vi "Digital Pattern Gen 1.3 In Place Settings Write Structure.vi"(5 "device inputs":dbl[](array[numeric]), 6 "device outputs in":dbl[](array[numeric]), 7 "last device inputs":dbl[](array[numeric]), 8 "error in (no error)":errorcluster, 9 "FPGA ref in":T1, 11 "1.3 digital pattern gen in":T2) -> (0 "error out":errorcluster, 1 "FPGA ref out":T1, 3 "1.3 digital pattern gen out":T2, 4 "device outputs out":dbl[](array[numeric]))   [LabVIEW 2019, in "Engine Simulation Toolkit Engine.lvlib"]
uses:
  Engine Simulation Toolkit Engine.lvlib
  Shared/1.3 Digital Pattern Gen Engine Data.ctl
  Shared/1.3 Digital Pattern Gen FIFO Idxs.ctl
  Digital Pattern Gen 1.3 Settings Ref.ctl
  Shared/Engine Simulation Toolkit Shared.lvlib
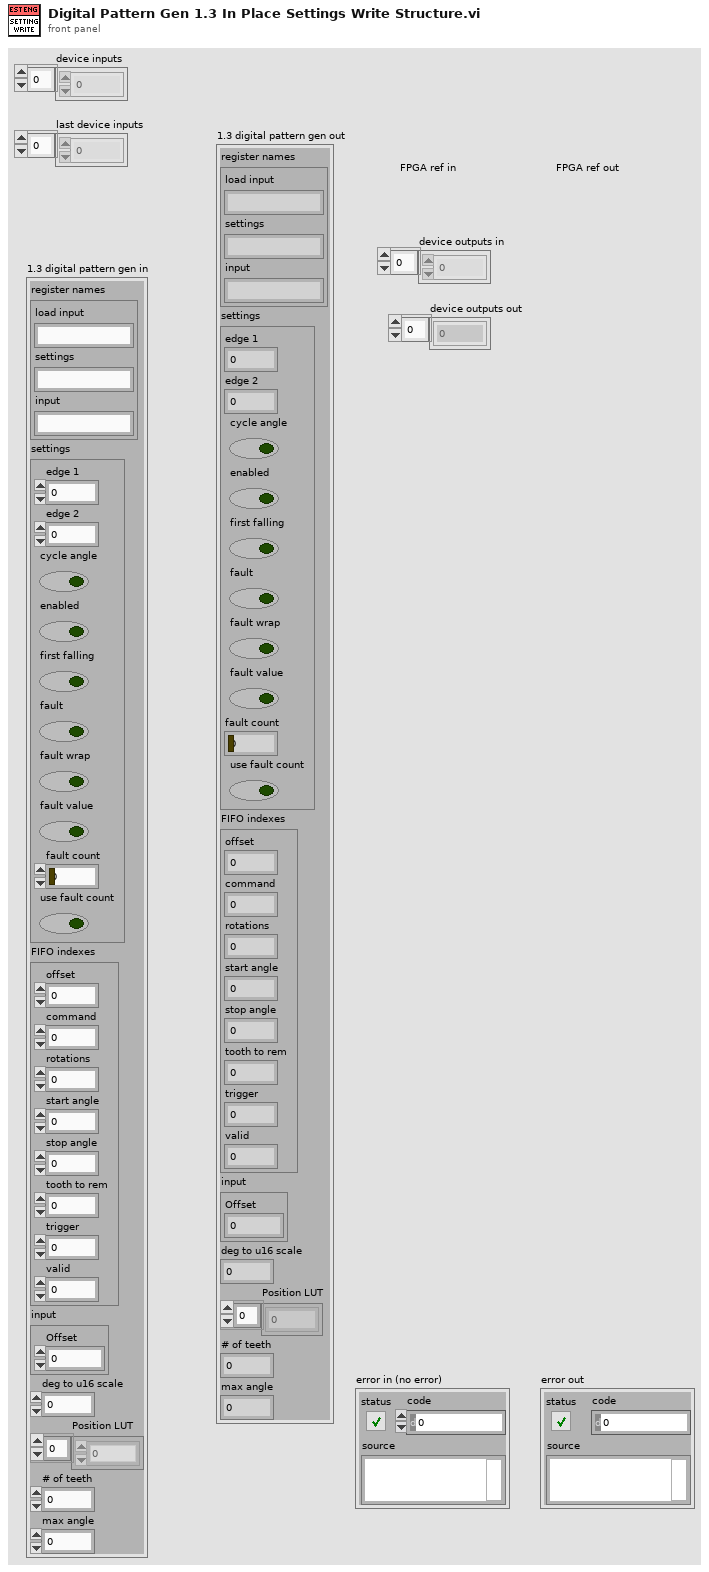
[diagram p1: front panel]
types:
  T1 = typedef "Engine Simulation Toolkit Engine.lvlib/Digital Pattern Gen 1.3 Settings Ref.ctl" = refnum<k20>
  T2 = typedef "Engine Simulation Toolkit Shared.lvlib/1.3 Digital Pattern Gen Engine Data.ctl" = cluster{"register names":cluster{"load input":string, "settings":string, "input":string}, "settings":cluster{"edge 1":u16, "edge 2":u16, "cycle angle":bool, "enabled":bool, "first falling":bool, "fault":bool, "fault wrap":bool, "fault value":bool, "fault count":fxp<+,4,4>, "use fault count":bool}, "FIFO indexes":T3, "input":cluster{"Offset":i16}, "deg to u16 scale":dbl, "Position LUT":u16[], "# of teeth":i16, "max angle":dbl}
  T3 = typedef "Engine Simulation Toolkit Shared.lvlib/1.3 Digital Pattern Gen FIFO Idxs.ctl" = cluster{"offset":i32, "command":i32, "rotations":i32, "start angle":i32, "stop angle":i32, "tooth to rem":i32, "trigger":i32, "valid":i32}
  T4 = cluster{"edge 1":u16, "edge 2":u16, "cycle angle":bool, "enabled":bool, "first falling":bool, "fault":bool, "fault wrap":bool, "fault value":bool, "fault count":fxp<+,4,4>, "use fault count":bool}
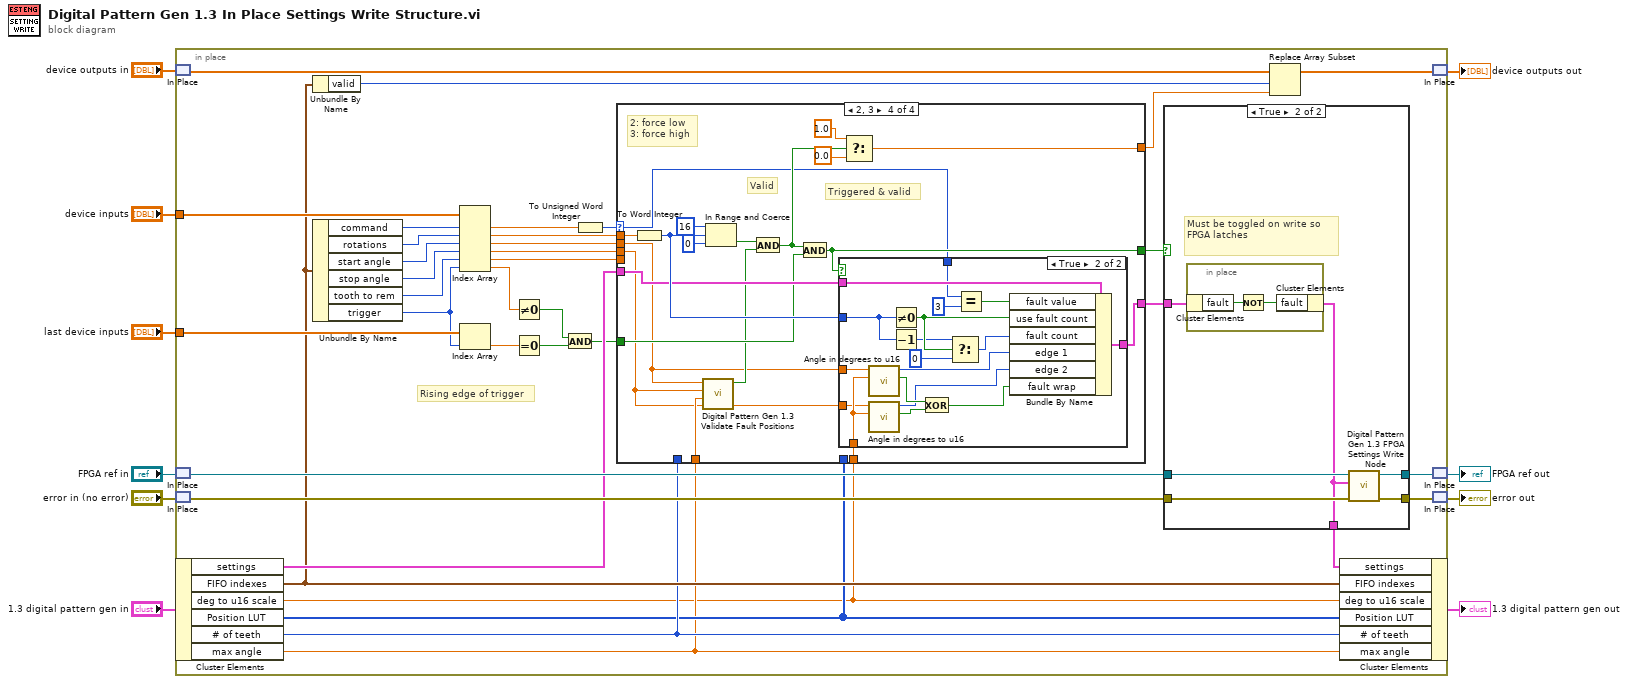
[diagram p0: block diagram]
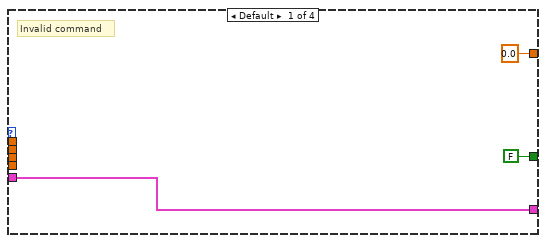
[diagram p3: hidden frame]
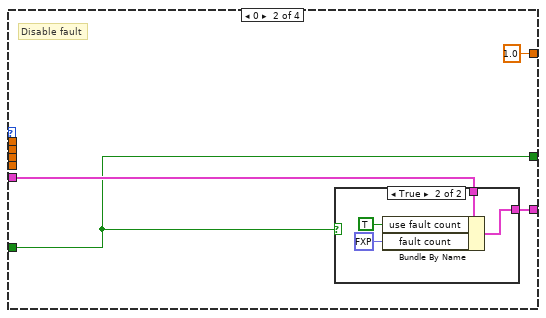
[diagram p4: hidden frame]
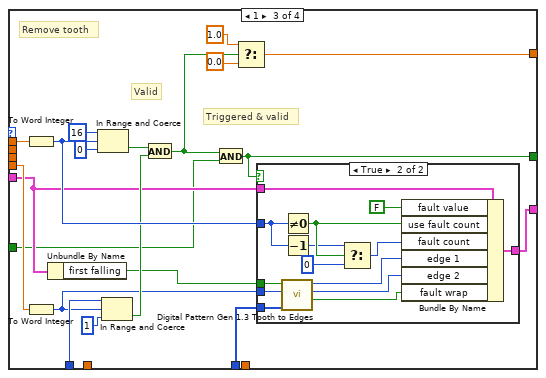
[diagram p6: hidden frame]
diagram:
  n1 = in-place {
    in-place-border: "device inputs" -> [w45]
    in-place-border: "last device inputs" -> [w44]
    # "Rising edge of trigger"
    n2 = in-place-match #1("device outputs in") -> (w46:dbl[])
    n3 = in-place-match #2("FPGA ref in") -> (w35:T1)
    n4 = in-place-match #3("error in (no error)") -> (w34:errorcluster)
    n5 = in-place-cluster #4("1.3 digital pattern gen in") -> ("settings"=w23:T4, "FIFO indexes"=w19:T3, "deg to u16 scale"=w11:dbl, "Position LUT"=w14:u16[], "# of teeth"=w17:i16, "max angle"=w12:dbl)
    n6 = Unbundle By Name(w19) -> ("valid"=w18:i32)
    n7 = Unbundle By Name(w19) -> ("command"=w43:i32, "rotations"=w42:i32, "start angle"=w41:i32, "stop angle"=w40:i32, "tooth to rem"=w39:i32, "trigger"=w38:i32)
    n8 = Index Array(array=w45, index #1=w43, index #2=w42, index #3=w41, index #4=w40, index #5=w39, index #6=w38) -> (element #1=w32:dbl, element #2=w31:dbl, element #3=w30:dbl, element #4=w29:dbl, element #5=w28:dbl, element #6=w21:dbl)
    n9 = Index Array(array=w44, index=w38) -> (element=w20:dbl)
    n10 = Not Equal To 0?(x=w21) -> (x != 0?=w25:bool)
    n11 = Equal To 0?(x=w20) -> (x = 0?=w24:bool)
    n12 = And(x=w25, y=w24) -> (x .and. y?=w15:bool)
    n13 = To Unsigned Word Integer(number=w32) -> (unsigned 16bit integer=w27:u16)
    n14 = case shown="2, 3" w27 {
      selector: w27 -> [_ _ _ w108]
      tunnel: w31 -> [_ _ w86 w120]
      tunnel: w30 -> [_ _ _ w105]
      tunnel: w29 -> [_ _ _ w106]
      tunnel: w28 -> [_ _ w82 _]
      tunnel: [FALSE w61 w73 w111] -> w16
      tunnel: [0.0 1.0 w83 w117] -> w26
      tunnel: w23 -> [w60 w63 w76 w114]
      tunnel: [w60 w62 w89 w123] -> w22
      tunnel: w17 -> [_ _ w80 _]
      tunnel: w15 -> [_ w61 w74 w112]
      tunnel: w14 -> [_ _ w70 _]
      tunnel: w12 -> [_ _ _ w110]
      tunnel: w11 -> [_ _ _ w107]
      frame Default {
        # "Invalid command"
      }
      frame 0 {
        # "Disable fault"
        n15 = case shown="True" w61 {
          tunnel: w63 -> [w65 w69]
          tunnel: [w65 w68] -> w62
          frame False {
          }
          frame True {
            n16 = Bundle By Name(cluster=w69, "use fault count"=TRUE, "fault count"=fxp<+,4,4> 0.0) -> (w68:T4)
          }
        }
      }
      frame 1 {
        # "Triggered & valid"
        # "Valid"
        # "Remove tooth"
        n17 = To Word Integer(number=w86) -> (16bit integer=w79:i16)
        n18 = To Word Integer(number=w82) -> (16bit integer=w71:i16)
        n19 = Unbundle By Name(w76) -> ("first falling"=w72:bool)
        n20 = In Range and Coerce(upper limit=i16 16, x=w79, lower limit=i16 0) -> (In Range?=w78:bool)  [unwired: 1 out]
        n21 = In Range and Coerce(upper limit=w80, x=w71, lower limit=i16 1) -> (In Range?=w77:bool)  [unwired: 1 out]
        n22 = And(x=w78, y=w77) -> (x .and. y?=w75:bool)
        n23 = And(x=w75, y=w74) -> (x .and. y?=w73:bool)
        n24 = Select(t=1.0, s=w75, f=0.0) -> (s? t:f=w83:dbl)
        n25 = case shown="True" w73 {
          tunnel: [w90 w104] -> w89
          tunnel: w79 -> [_ w102]
          tunnel: w76 -> [w90 w98]
          tunnel: w72 -> [_ w96]
          tunnel: w71 -> [_ w95]
          tunnel: w70 -> [_ w94]
          frame False {
          }
          frame True {
            n26 = call "Digital Pattern Gen 1.3 Tooth to Edges.vi"("position LUT"=w94, "tooth to remove"=w95, "first falling"=w96) -> ("fault wrap"=w91:bool, "edge 2"=w92:u16, "edge 1"=w93:u16)  [unwired: 6 in]
            n27 = Not Equal To 0?(x=w102) -> (x != 0?=w103:bool)
            n28 = Decrement(x=w102) -> (x-1=w101:i16)
            n29 = Select(t=w101, s=w103, f=i16 0) -> (s? t:f=w100:i16)
            n30 = Bundle By Name(cluster=w98, "fault value"=FALSE, "use fault count"=w103, "fault count"=w100, "edge 1"=w93, "edge 2"=w92, "fault wrap"=w91) -> (w104:T4)
          }
        }
      }
      frame 2, 3 {
        # "Triggered & valid"
        # "Valid"
        # "2: force low\n3: force high"
        n31 = To Word Integer(number=w120) -> (16bit integer=w116:i16)
        n32 = call "Digital Pattern Gen 1.3 Validate Fault Positions.vi"("max angle"=w110, "end angle"=w106, "start angle"=w105) -> ("valid"=w109:bool)  [unwired: 8 in]
        n33 = In Range and Coerce(upper limit=i16 16, x=w116, lower limit=i16 0) -> (In Range?=w115:bool)  [unwired: 1 out]
        n34 = And(x=w115, y=w109) -> (x .and. y?=w113:bool)
        n35 = And(x=w113, y=w112) -> (x .and. y?=w111:bool)
        n36 = case shown="True" w111 {
          tunnel: [w124 w142] -> w123
          tunnel: w116 -> [_ w140]
          tunnel: w114 -> [w124 w136]
          tunnel: w108 -> [_ w135]
          tunnel: w107 -> [_ w127]
          tunnel: w106 -> [_ w126]
          tunnel: w105 -> [_ w125]
          frame False {
          }
          frame True {
            n37 = call "Angle in degrees to u16.vi"("angle to u16 scale factor"=w127, "Angle (deg)"=w125) -> ("angle < 0?"=w132:bool, "u16 angle"=w128:u16)  [unwired: 8 in]
            n38 = call "Angle in degrees to u16.vi"("angle to u16 scale factor"=w127, "Angle (deg)"=w126) -> ("angle < 0?"=w131:bool, "u16 angle"=w129:u16)  [unwired: 8 in]
            n39 = Not Equal To 0?(x=w140) -> (x != 0?=w141:bool)
            n40 = Decrement(x=w140) -> (x-1=w139:i16)
            n41 = Exclusive Or(1:w131, 2:w132) -> (0:w130:bool)
            n42 = Select(t=w139, s=w141, f=i16 0) -> (s? t:f=w138:i16)
            n43 = Equal?(x=w135, y=u16 3) -> (x = y?=w133:bool)
            n44 = Bundle By Name(cluster=w136, "fault value"=w133, "use fault count"=w141, "fault count"=w138, "edge 1"=w128, "edge 2"=w129, "fault wrap"=w130) -> (w142:T4)
          }
        }
        n45 = Select(t=1.0, s=w113, f=0.0) -> (s? t:f=w117:dbl)
      }
    }
    n46 = case shown="True" w16 {
      tunnel: [w49 w53] -> w36
      tunnel: w35 -> [w49 w55]
      tunnel: w34 -> [w48 w52]
      tunnel: [w48 w54] -> w33
      tunnel: w22 -> [w47 w51]
      tunnel: [w47 w50] -> w13
      frame False {
      }
      frame True {
        # "Must be toggled on write so FPGA latches"
        n47 = in-place {
          n48 = in-place-cluster #5(w51) -> ("fault"=w57:bool)
          n49 = Not(x=w57) -> (.not. x?=w56:bool)
          n50 = in-place-cluster #5("fault"=w56) -> (w50:T4)
        }
        n51 = call "Digital Pattern Gen 1.3 FPGA Settings Write Node.vi"("error in (no error)"=w52, "settings"=w50, "Refnum in"=w55) -> ("error out"=w54:errorcluster, "Refnum out"=w53:T1)  [unwired: 7 in]
      }
    }
    n52 = Replace Array Subset(array=w46, new element=w26, index=w18) -> (w37:dbl[])
    n53 = in-place-cluster #4("settings"=w13, "FIFO indexes"=w19, "deg to u16 scale"=w11, "Position LUT"=w14, "# of teeth"=w17, "max angle"=w12) -> (→"1.3 digital pattern gen out":T2)
    n54 = in-place-match #1(w37) -> (→"device outputs out":dbl[])
    n55 = in-place-match #2(w36) -> (→"FPGA ref out":T1)
    n56 = in-place-match #3(w33) -> (→"error out":errorcluster)
  }
